vi "Config ACTION.vi"(8 "error in (no error)":errorcluster, 11 "AutoZero in":refnum<class "AutoZero.lvclass">) -> (0 "error out":errorcluster, 3 "AutoZero out":refnum<class "AutoZero.lvclass">)   [LabVIEW 2014, in "SeqLoop.lvlib" / "STEP Classes.lvlib" / "AutoZero.lvclass"]
uses:
  AutoZero.lvclass
  Resources/XControls/Selectable ListBox xControl/ListBox XControl.xctl
  <vilib>/Utility/miscctls.llb/LVPointTypeDef.ctl
  AutoZero.lvclass/AutoZero.ctl
panel:
  in  "AutoZero HWAsync?":T1
  in  "Deselect All":bool
  in  "Select All":bool
  in  "Cancel":bool
  in  "Save":bool
  in  "Measurement List":string[](xcontrol)
  # "Seleccione Transductores para Cerar"
  # "Hardware Asíncronos"
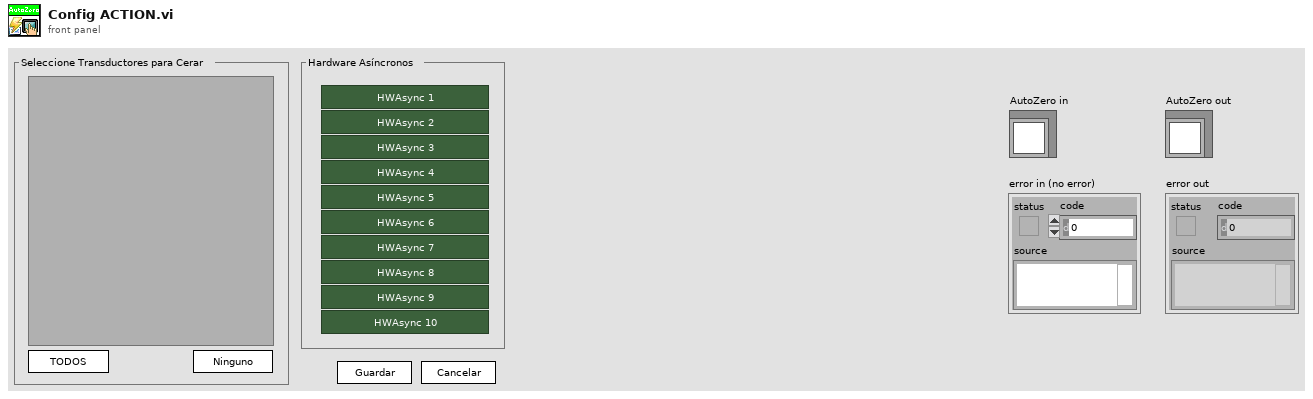
[diagram p1: front panel]
types:
  T1 = cluster{"HWAsync 1":bool, "HWAsync 2":bool, "HWAsync 3":bool, "HWAsync 4":bool, "HWAsync 5":bool, "HWAsync 6":bool, "HWAsync 7":bool, "HWAsync 8":bool, "HWAsync 9":bool, "HWAsync 10":bool}
  T2 = typedef "LVPointTypeDef.ctl" = cluster{"Horizontal":i16, "Vertical":i16}
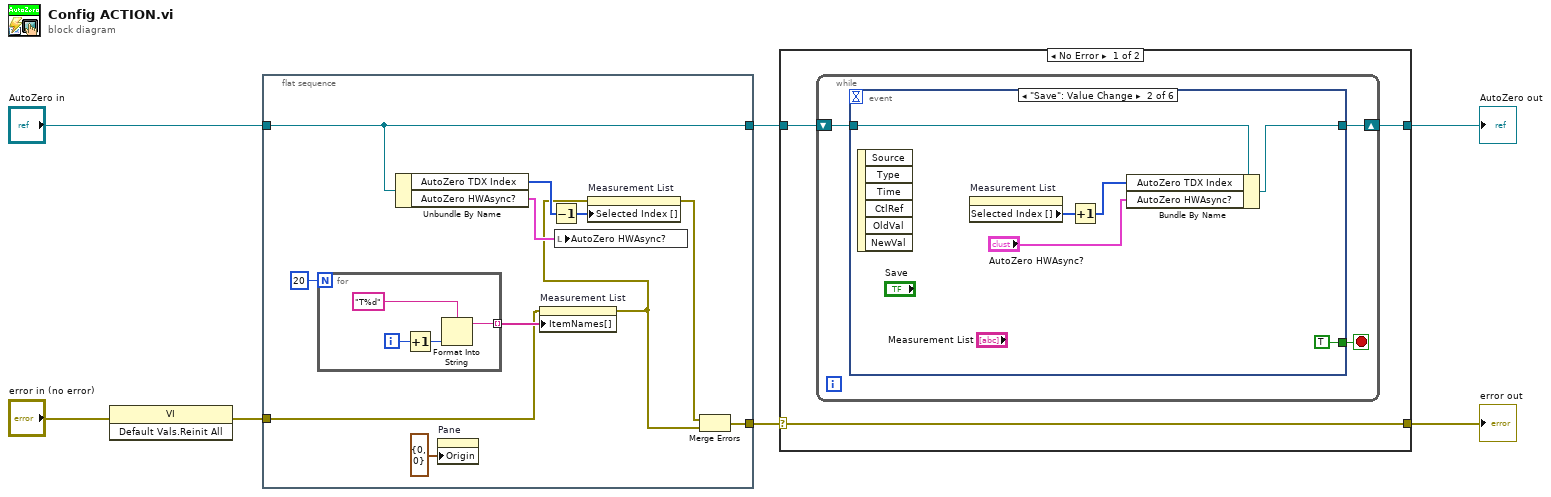
[diagram p0: block diagram]
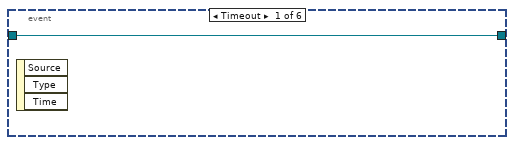
[diagram p2: hidden frame]
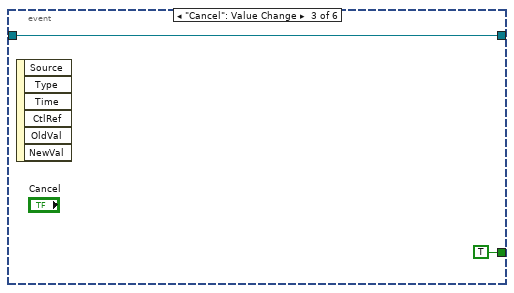
[diagram p3: hidden frame]
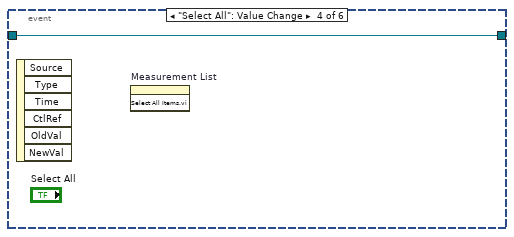
[diagram p4: hidden frame]
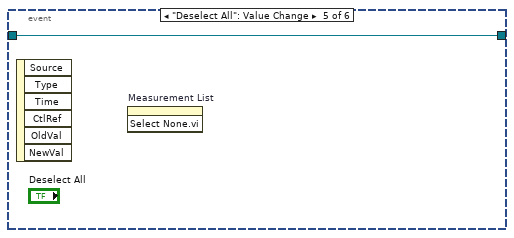
[diagram p5: hidden frame]
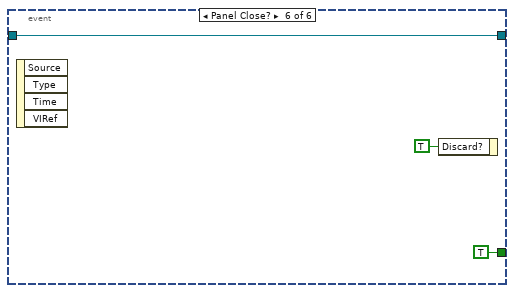
[diagram p6: hidden frame]
diagram:
  n1 = invoke class="VI" method="Default Vals.Reinit All"(error in="error in (no error)") -> (error out=w6:errorcluster)  [unwired: 2 in, 2 out]
  n2 = flat-sequence {
    tunnel: "AutoZero in" -> [w11]
    tunnel: [w15] -> w7
    tunnel: w6 -> [w9]
    tunnel: [w11] -> w5
    frame #0 {
      n3 = for {
        N: 20 -> [_]
        tunnel: [w19] -> w18 mode=indexing
        i -> [w20]
        n4 = Increment(x=w20) -> (x+1=w21:i32)
        n5 = Format Into String(format string="T%d", w21) -> (resulting string=w19:string)  [unwired: 2 in, 1 out]
      }
      n6 = Unbundle By Name(w11) -> ("AutoZero TDX Index"=w12:i32[], "AutoZero HWAsync?"=w16:T1)
      n7 = property on="Pane" class="Pane"("Origin"=T2 {"Horizontal"=0, "Vertical"=0}) -> ()  [unwired: 2 in, 2 out]
      n8 = property on="Measurement List" class="ListBox XControl (strict)"(error in=w9, "ItemNames[]"=w18) -> (error out=w8:errorcluster)  [unwired: 1 in, 1 out]
      n9 = Decrement(x=w12) -> (x-1=w13:i32[])
      n10 = local write "AutoZero HWAsync?"(w16) -> ()
      n11 = property on="Measurement List" class="ListBox XControl (strict)"(error in=w8, "Selected Index []"=w13) -> (error out=w14:errorcluster)  [unwired: 1 in, 1 out]
      n12 = Merge Errors(w14, w8) -> (w15:errorcluster)
    }
  }
  n13 = case shown="No Error" w7 {
    selector: w7 -> [w25 w44]
    tunnel: [w25 w44] -> w2
    tunnel: [w23 w43] -> w3
    tunnel: w5 -> [w24 w43]
    frame No Error {
      n14 = while {
        shift-right: [w27] -> w23
        shift-left: w24 -> [w28]
        stop <- w26 stop-if-true
        n15 = event shown="[1] \"Save\": Value Change" {
          selector: _ -> [_ _ _ _ _ _]
          dyn-events: _ -> [_ _ _ _ _ _]
          timeout: _ -> [_ _ _ _ _ _]
          tunnel: w28 -> [w29 w34 w37 w38 w39 w42]
          tunnel: [w29 w33 w37 w38 w39 w42] -> w27
          tunnel: [_ TRUE TRUE _ _ TRUE] -> w26
          event Timeout {
            n16 = event-data() -> ()  [unwired: 1 in, 3 out]
          }
          event "Save": Value Change {
            n17 = event-data() -> ()  [unwired: 1 in, 6 out]
            n18 = property on="Measurement List" class="ListBox XControl (strict)"() -> ("Selected Index []"=w32:i32[])  [unwired: 2 in, 2 out]
            n19 = Increment(x=w32) -> (x+1=w31:i32[])
            n20 = Bundle By Name(cluster=w34, "AutoZero TDX Index"=w31, "AutoZero HWAsync?"="AutoZero HWAsync?") -> (w33:refnum<class "AutoZero.lvclass">)
          }
          event "Cancel": Value Change {
            n21 = event-data() -> ()  [unwired: 1 in, 6 out]
          }
          event "Select All": Value Change {
            n22 = event-data() -> ()  [unwired: 1 in, 6 out]
            n23 = invoke on="Measurement List" class="ListBox XControl (strict)" method="Select All Items.vi"() -> ()  [unwired: 3 in, 3 out]
          }
          event "Deselect All": Value Change {
            n24 = event-data() -> ()  [unwired: 1 in, 6 out]
            n25 = invoke on="Measurement List" class="ListBox XControl (strict)" method="Select None.vi"() -> ()  [unwired: 3 in, 3 out]
          }
          event Panel Close? {
            n26 = event-data() -> ()  [unwired: 1 in, 4 out]
            n27 = event-data("Discard?"=TRUE) -> ()  [unwired: 1 in, 1 out]
          }
        }
      }
    }
    frame Error {
    }
  }
  "error out" <- w2
  "AutoZero out" <- w3
